vi "Send to Redlines.vi"(8 "error in (no error)":errorcluster, 10 "Data":T1, 11 "Data Processor Module in":refnum<class "Data Processor Module.lvclass">) -> (0 "error out":errorcluster, 2 "Data dup":T1, 3 "Data Processor Module out":refnum<class "Data Processor Module.lvclass">)   [LabVIEW 2020, in "VolatusData.lvlib" / "Data Processor Module.lvclass"]
uses:
  Data Processor Module.lvclass
  Data Processor Module.lvclass/Data Processor Module.ctl
  Volatus/MessageQ/MessageQ.lvclass
  New Data.ctl
  VolatusData.lvlib
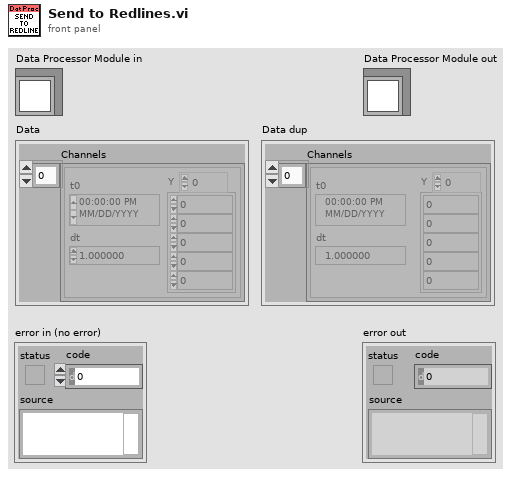
[diagram p1: front panel]
types:
  T1 = typedef "VolatusData.lvlib/New Data.ctl" = cluster{"Channels":waveform(dbl)[]}
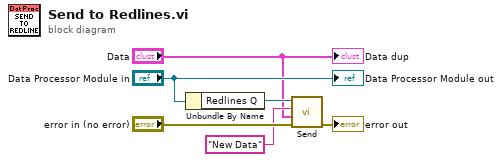
[diagram p0: block diagram]
diagram:
  n1 = Unbundle By Name("Data Processor Module in") -> ("Redlines Q"=w4:refnum<class "MessageQ.lvclass">)
  n2 = call "Send.vi"("error in (no error)"="error in (no error)", "Data"="Data", "ID"="New Data", "MessageQ in"=w4) -> ("error out"=→"error out":errorcluster)  [unwired: 6 in, 1 out]
  "Data Processor Module out" <- "Data Processor Module in"
  "Data dup" <- "Data"
